vi "Write reference.vi"(8 "error in (no error)":errorcluster, 10 "reference":refnum<k24>, 11 "MelsecTCP in":refnum<class "Inovance5UTcp.lvclass">) -> (0 "error out":errorcluster, 3 "MelsecTCP out":refnum<class "Inovance5UTcp.lvclass">)   [LabVIEW 2020, in "HslCommunication.lvlib" / "Inovance5UTcp.lvclass"]
uses:
  Inovance5UTcp.lvclass
  D:/Git/Labview-Libraries/builds/HslCommunication/HslCommunication.dll
  builds/HslCommunication/HslCommunication.dll
  Inovance5UTcp.lvclass/Inovance5UTcp.ctl
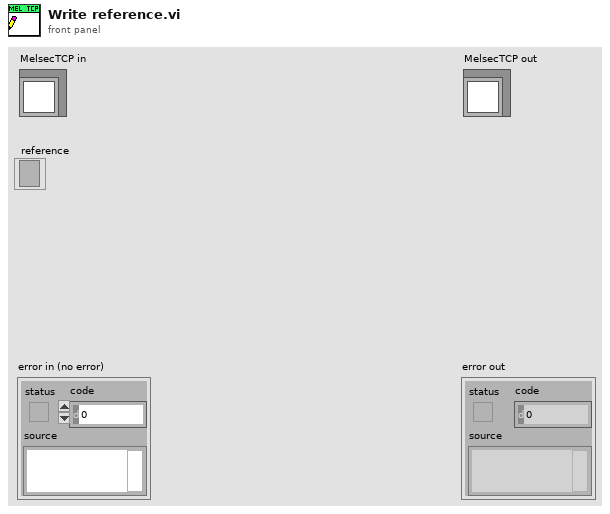
[diagram p1: front panel]
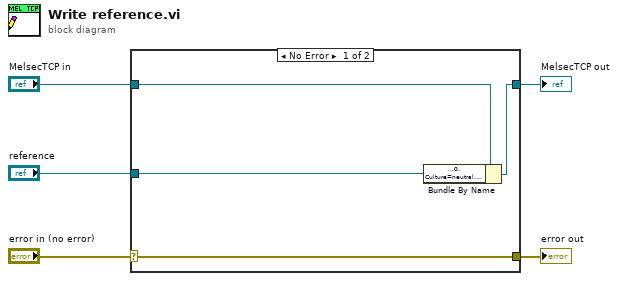
[diagram p0: block diagram]
diagram:
  n1 = case shown="No Error" "error in (no error)" {
    selector: "error in (no error)" -> [w9 w10]
    tunnel: [w9 w10] -> w4
    tunnel: [w7 w11] -> w2
    tunnel: "MelsecTCP in" -> [w8 w11]
    tunnel: "reference" -> [w6 _]
    frame No Error {
      n2 = Bundle By Name(cluster=w8, "reference"=w6) -> (w7:refnum<class "Inovance5UTcp.lvclass">)
    }
    frame Error {
    }
  }
  "error out" <- w4
  "MelsecTCP out" <- w2
